vi "Write Acquire Pulse Ref.vi"(8 "error in (no error)":errorcluster, 10 "Acquire Pulse Ref":refnum<vi>, 11 "Measure Pulse in":refnum<class "Measure Pulse.lvclass">) -> (0 "error out":errorcluster, 3 "Measure Pulse out":refnum<class "Measure Pulse.lvclass">)   [LabVIEW 2015, in "Measure Pulse.lvclass"]
uses:
  Measure Pulse.lvclass
  Queued Listbox/Queued Listbox.xctl
  Measure Pulse.lvclass/Measure Pulse.ctl
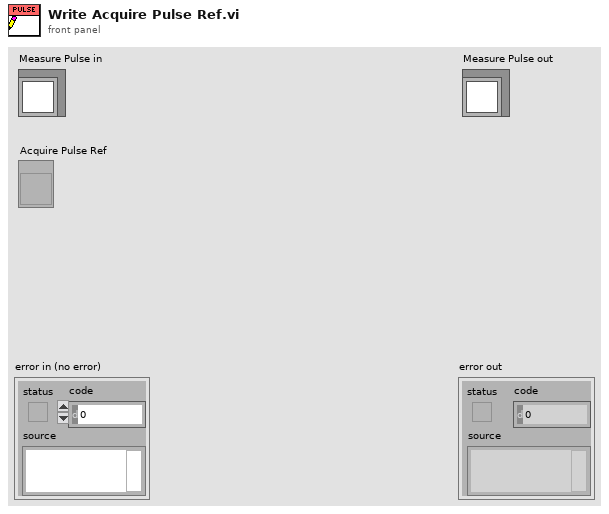
[diagram p1: front panel]
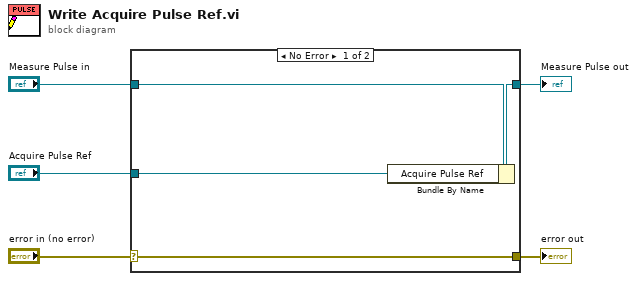
[diagram p0: block diagram]
diagram:
  n1 = case shown="No Error" "error in (no error)" {
    selector: "error in (no error)" -> [w9 w10]
    tunnel: [w9 w10] -> w4
    tunnel: [w7 w11] -> w2
    tunnel: "Measure Pulse in" -> [w8 w11]
    tunnel: "Acquire Pulse Ref" -> [w6 _]
    frame No Error {
      n2 = Bundle By Name(cluster=w8, "Acquire Pulse Ref"=w6) -> (w7:refnum<class "Measure Pulse.lvclass">)
    }
    frame Error {
    }
  }
  "error out" <- w4
  "Measure Pulse out" <- w2
